vi "Initiate Connection.vi"(8 "error in (no error)":errorcluster, 10 "Controller Address":string) -> (0 "error out":errorcluster, 2 "writer endpoint":refnum<k21>, 3 "reader endpoint":refnum<k21>)   [LabVIEW 2015, in "Tool Interface.lvlib"]
uses:
  Tool Interface.lvlib
  Tool Typedefs/Message Cluster.ctl
  GLOB - Configuration Options.vi
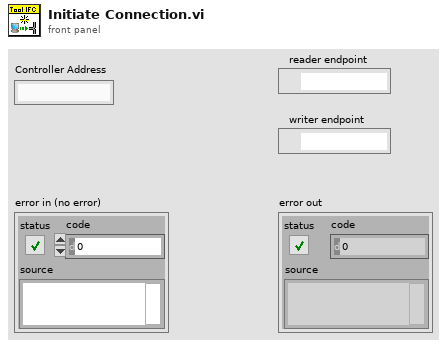
[diagram p1: front panel]
types:
  T1 = typedef "Message Cluster.ctl" = cluster{"Message":string, "Message Data":variant}
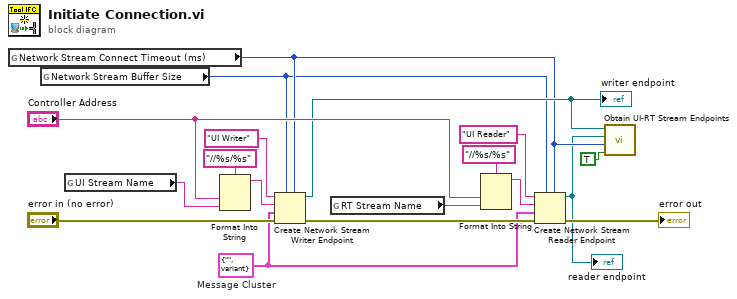
[diagram p0: block diagram]
diagram:
  w8 = T1 {"Message"="", "Message Data"=variant}  # Message Cluster
  n1 = global read "GLOB - Configuration Options.vi" "Network Stream Connect Timeout (ms)"() -> (w3:i32)
  n2 = global read "GLOB - Configuration Options.vi" "Network Stream Buffer Size"() -> (w2:i32)
  n3 = global read "GLOB - Configuration Options.vi" "UI Stream Name"() -> (w9:string)
  n4 = Format Into String(format string="//%s/%s", "Controller Address", w9) -> (resulting string=w15:string)  [unwired: 2 in, 1 out]
  n5 = Create Network Stream Writer Endpoint(5:w3, 7:w2, 8:"error in (no error)", 9:w8, 10:w15, 11:"UI Writer" ("reader name")) -> (0:w18:errorcluster, 3:w5:refnum<k21>)  [unwired: 1 in]
  "writer endpoint" <- w5
  n6 = global read "GLOB - Configuration Options.vi" "RT Stream Name"() -> (w10:string)
  n7 = Format Into String(format string="//%s/%s", "Controller Address", w10) -> (resulting string=w13:string)  [unwired: 2 in, 1 out]
  n8 = Create Network Stream Reader Endpoint(5:w3, 7:w2, 8:w18, 9:w8, 10:w13, 11:"UI Reader" ("writer name")) -> (0:→"error out":errorcluster, 3:w1:refnum<k21>)  [unwired: 1 in]
  "reader endpoint" <- w1
  n9 = call "Obtain UI-RT Stream Endpoints.vi"("New"=TRUE, "Connect Timeout(ms) in"=w3, "reader endpoint"=w1, "writer endpoint"=w5) -> ()  [unwired: 5 in, 3 out]
